vi "Analysis_simple_worker.vi"(5 "Leftover data in":T1, 6 "error in":errorcluster, 7 "Pixels to integrate":i32, 8 "Data in":T1) -> (0 "error out":errorcluster, 2 "Data out":T1, 4 "Leftover data out":T1)   [LabVIEW 2010]
uses:
  typedefs/data_cluster.ctl
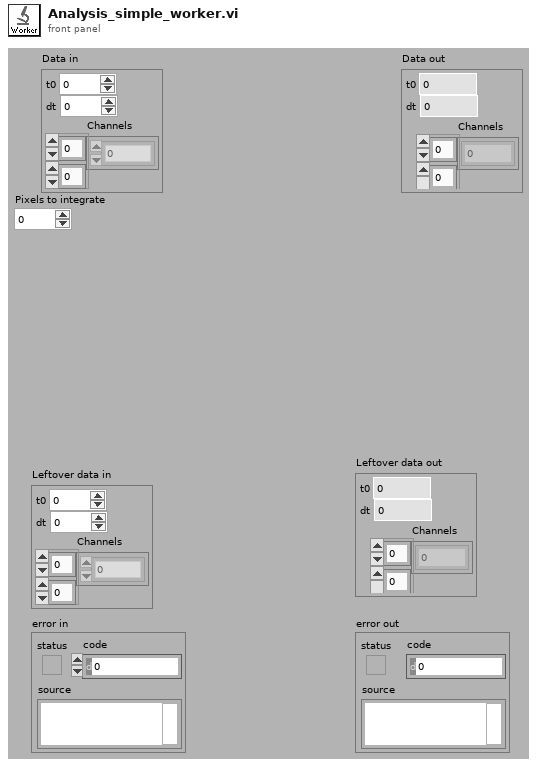
[diagram p1: front panel]
types:
  T1 = typedef "data_cluster.ctl" = cluster{"t0":dbl, "dt":dbl, "Channels":dbl[][]}
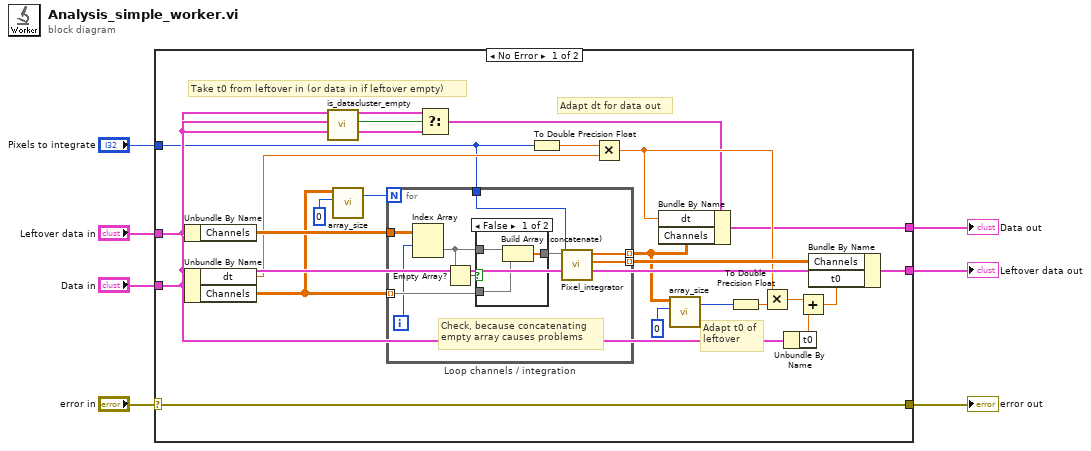
[diagram p0: block diagram]
diagram:
  n1 = case shown="No Error" "error in" {
    selector: "error in" -> [w24 w46]
    tunnel: "Data in" -> [w21 w45]
    tunnel: [w12 w45] -> w3
    tunnel: "Leftover data in" -> [w22 w44]
    tunnel: [w25 w44] -> w4
    tunnel: [w24 w46] -> w2
    tunnel: "Pixels to integrate" -> [w13 _]
    frame No Error {
      # "Adapt t0 of\nleftover"
      # "Adapt dt for data out"
      # "Take t0 from leftover in (or data in if leftover empty)"
      n2 = Unbundle By Name(w22) -> ("Channels"=w30:dbl[][])
      n3 = Unbundle By Name(w21) -> ("dt"=w18:dbl, "Channels"=w15:dbl[][])
      n4 = call "is_datacluster_empty.vi"("Data_cluster"=w22) -> ("Is empty?"=w23:bool)  [unwired: 10 in]
      n5 = call "array_size.vi"("Array"=w15, "Dimension"=0) -> ("Dimension size"=w14:i32)  [unwired: 4 in]
      n6 = for "Loop channels / integration" {
        N: w14 -> [_]
        tunnel: w13 -> [w39]
        tunnel: [w35] -> w10 mode=indexing
        tunnel: [w38] -> w29 mode=indexing
        tunnel: w15 -> [w37] mode=indexing
        tunnel: w30 -> [w33]
        i -> [w31]
        # "Check, because concatenating\nempty array causes problems"
        n7 = Index Array(array=w33, index (row)=w31) -> (element=w32:dbl[])  [unwired: 1 in]
        n8 = Empty Array?(array=w32) -> (empty?=w34:bool)
        n9 = case shown="False" w34 {
          tunnel: w32 -> [w42 _]
          tunnel: w37 -> [w41 w43]
          tunnel: [w40 w43] -> w36
          frame False {
            n10 = Build Array (concatenate)(w42, w41) -> (w40:dbl[])
          }
          frame True {
          }
        }
        n11 = call "Pixel_integrator.vi"("Pixels to integrate"=w39, "Data in"=w36) -> ("Leftover data out"=w38:dbl[], "Data out"=w35:dbl[])  [unwired: 6 in]
      }
      n12 = Select(t=w21, s=w23, f=w22) -> (s? t:f=w17:T1)
      n13 = To Double Precision Float(number=w13) -> (double precision float=w16:dbl)
      n14 = Multiply(x=w16, y=w18) -> (x*y=w19:dbl)
      n15 = Bundle By Name(cluster=w17, "dt"=w19, "Channels"=w10) -> (w12:T1)
      n16 = call "array_size.vi"("Array"=w10, "Dimension"=0) -> ("Dimension size"=w9:i32)  [unwired: 4 in]
      n17 = To Double Precision Float(number=w9) -> (double precision float=w20:dbl)
      n18 = Multiply(x=w19, y=w20) -> (x*y=w28:dbl)
      n19 = Unbundle By Name(w21) -> ("t0"=w27:dbl)
      n20 = Add(x=w28, y=w27) -> (x+y=w26:dbl)
      n21 = Bundle By Name(cluster=w21, "Channels"=w29, "t0"=w26) -> (w25:T1)
    }
    frame Error {
    }
  }
  "error out" <- w2
  "Data out" <- w3
  "Leftover data out" <- w4
